vi "SRX_Config_Set Limit Travel Values.vi"(6 "Send Cmd Timout(ms)":u32, 8 "Error":errorcluster, 9 "Limits":T6 {"Soft"."REV"."Counts" format="%#.0f"; "Soft"."FWD"."Counts" format="%#.0f"}, 11 "PhoenixMotorControlDevRef":T1) -> (0 "Error Out":errorcluster, 3 "PhoenixMotorControlDevRef Out":T1)   [LabVIEW 2020]
uses:
  Shared Code/TypeDefs/Cluser_Limit Travel Config.ctl
  Shared Code/TypeDefs/Cluser_Hard Limits.ctl
  <vilib>/Rock Robotics/WPI/ThirdParty/Phoenix-LabVIEW/Motor Controller/Controls/CTRE_Phoenix_MotorControl_LimitSwitchNormal.ctl
  Shared Code/TypeDefs/Cluser_Config_Soft Limits.ctl
  Shared Code/TypeDefs/Cluser_Enable-Value I32.ctl
  <vilib>/Rock Robotics/WPI/MotorControl/WPI_MotorControlDeviceRef.ctl
  <vilib>/Rock Robotics/WPI/MotorControl/WPI_MotorControlType.ctl
  <vilib>/Rock Robotics/SystemInterfaces/DIO/FPGA_DIOPWMChannel.ctl
  <vilib>/Rock Robotics/WPI/PWM/WPI_PWMDeadband.ctl
  <vilib>/Rock Robotics/SystemInterfaces/DIO/FPGA_DIOChannel.ctl
  <vilib>/Rock Robotics/WPI/ThirdParty/Phoenix-LabVIEW/Motor Controller/Controls/CTRE_Phoenix_MotorControl_LimitSwitchSource_Local.ctl
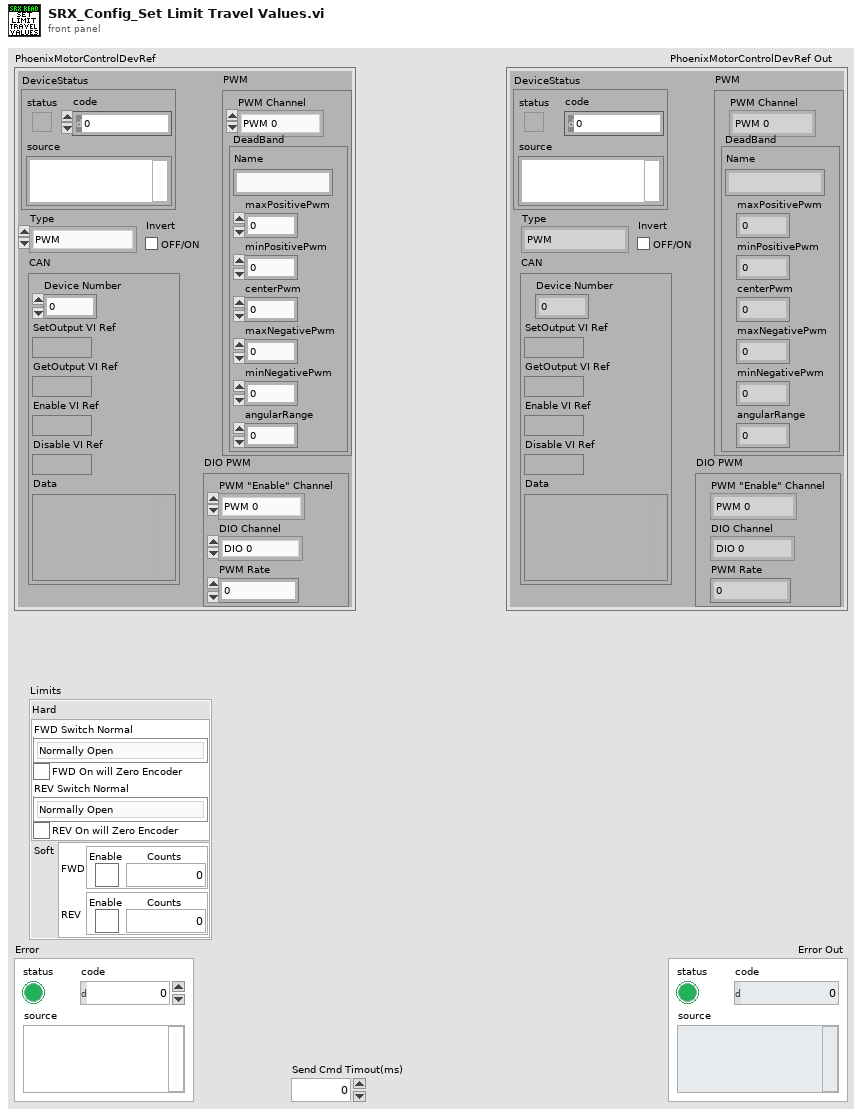
[diagram p1: front panel]
types:
  T1 = typedef "WPI_MotorControlDeviceRef.ctl" = cluster{"DeviceStatus":errorcluster, "Type":T2, "PWM":cluster{"PWM Channel":T3, "DeadBand":T4}, "CAN":cluster{"Device Number":u8, "SetOutput VI Ref":variant, "GetOutput VI Ref":variant, "Enable VI Ref":variant, "Disable VI Ref":variant, "Data":variant}, "Invert":bool, "DIO PWM":cluster{"PWM \"Enable\" Channel":T3, "DIOChannel":T5, "PWM Rate":dbl}}
  T2 = typedef "WPI_MotorControlType.ctl" = enum16{"PWM", "CAN", "DIO PWM"}
  T3 = typedef "FPGA_DIOPWMChannel.ctl" = enum8{"PWM 0", "PWM 1", "PWM 2", "PWM 3", "PWM 4", "PWM 5", "PWM 6", "PWM 7", "PWM 8", "PWM 9", "PWM MXP 0", "PWM MXP 1", "PWM MXP 2", "PWM MXP 3", "PWM MXP 4", "PWM MXP 5", "PWM MXP 6", "PWM MXP 7", "PWM MXP 8", "PWM MXP 9", "Invalid"}
  T4 = typedef "WPI_PWMDeadband.ctl" = cluster{"Name":string, "maxPositivePwm":i32, "minPositivePwm":i32, "centerPwm":i32, "maxNegativePwm":i32, "minNegativePwm":i32, "angularRange":u16}
  T5 = typedef "FPGA_DIOChannel.ctl" = enum8{"DIO 0", "DIO 1", "DIO 2", "DIO 3", "DIO 4", "DIO 5", "DIO 6", "DIO 7", "DIO 8", "DIO 9", "DIO MXP 0", "DIO MXP 1", "DIO MXP 2", "DIO MXP 3", "DIO MXP 4", "DIO MXP 5", "DIO MXP 6", "DIO MXP 7", "DIO MXP 8", "DIO MXP 9", "DIO MXP 10", "DIO MXP 11", "DIO MXP 12", "DIO MXP 13", "DIO MXP 14", "DIO MXP 15", "SPI Port CS1", "SPI Port CS2", "SPI Port CS3", "SPI Port MISO", "SPI Port MOSI", "Invalid"}
  T6 = typedef "Cluser_Limit Travel Config.ctl" = cluster{"Hard":T7, "Soft":T9}
  T7 = typedef "Cluser_Hard Limits.ctl" = cluster{"FWD Switch Normal":T8, "FWD On will Zero Encoder ":bool, "REV Switch Normal":T8, "REV On will Zero Encoder ":bool}
  T8 = typedef "CTRE_Phoenix_MotorControl_LimitSwitchNormal.ctl" = enum16{"Normally Open", "Normally Closed", "Disabled"}
  T9 = typedef "Cluser_Config_Soft Limits.ctl" = cluster{"FWD":T10, "REV":T10}
  T10 = typedef "Cluser_Enable-Value I32.ctl" = cluster{"Enable":bool, "Counts":i32}
  T11 = typedef "CTRE_Phoenix_MotorControl_LimitSwitchSource_Local.ctl" = enum16{"Feedback Connector", "Remote Talon SRX", "Remote CANifier", "Deactivated"}
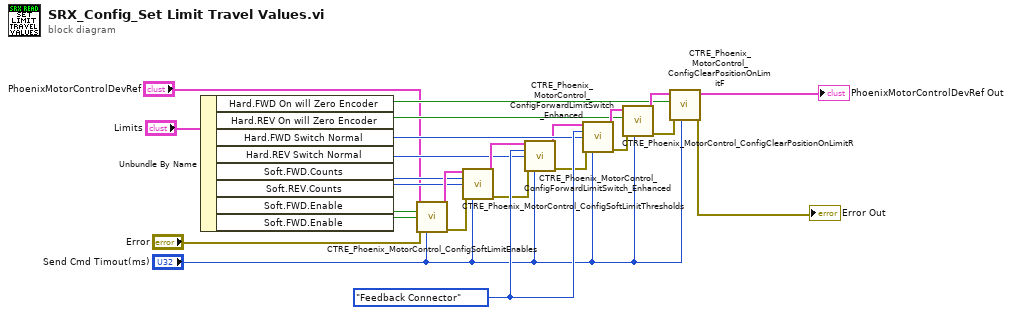
[diagram p0: block diagram]
diagram:
  w16 = CTRE_Phoenix_MotorControl_LimitSwitchSource_Local."Feedback Connector" ("Limit Switch Source")
  n1 = Unbundle By Name("Limits") -> ("Hard.FWD On will Zero Encoder"=w5:bool, "Hard.REV On will Zero Encoder"=w8:bool, "Hard.FWD Switch Normal"=w14:T8, "Hard.REV Switch Normal"=w15:T8, "Soft.FWD.Counts"=w19:i32, "Soft.REV.Counts"=w18:i32, "Soft.FWD.Enable"=w24:bool, "Soft.FWD.Enable"=w23:bool)
  n2 = call <vilib>:"CTRE_Phoenix_MotorControl_ConfigSoftLimitEnables.vi"("PhoenixMotorControlDevRef"="PhoenixMotorControlDevRef", "Forward Soft Limit Enable"=w24, "Reverse Soft Limit Enable"=w23, "error in (no error)"="Error", "timeoutMs"="Send Cmd Timout(ms)") -> ("PhoenixMotorControlDevRef"=w20:T1, "error out"=w21:errorcluster)  [unwired: 9 in]
  n3 = call <vilib>:"CTRE_Phoenix_MotorControl_ConfigSoftLimitThresholds.vi"("PhoenixMotorControlDevRef"=w20, "Forward Soft Limit"=w19, "Reverse Soft Limit"=w18, "error in (no error)"=w21, "timeoutMs"="Send Cmd Timout(ms)") -> ("PhoenixMotorControlDevRef"=w17:T1, "error out"=w12:errorcluster)  [unwired: 9 in]
  n4 = call <vilib>:"CTRE_Phoenix_MotorControl_ConfigForwardLimitSwitch_Enhanced.vi"("PhoenixMotorControlDevRef"=w17, "Limit Switch Source"=w16, "NormallyOpenOrClosed"=w15, "error in (no error)"=w12, "timeoutMs"="Send Cmd Timout(ms)") -> ("PhoenixMotorControlDevRef"=w11:T1, "error out"=w13:errorcluster)  [unwired: 9 in]
  n5 = call <vilib>:"CTRE_Phoenix_MotorControl_ConfigForwardLimitSwitch_Enhanced.vi"("PhoenixMotorControlDevRef"=w11, "Limit Switch Source"=w16, "NormallyOpenOrClosed"=w14, "error in (no error)"=w13, "timeoutMs"="Send Cmd Timout(ms)") -> ("PhoenixMotorControlDevRef"=w9:T1, "error out"=w10:errorcluster)  [unwired: 9 in]
  n6 = call <vilib>:"CTRE_Phoenix_MotorControl_ConfigClearPositionOnLimitR.vi"("timeoutMs"="Send Cmd Timout(ms)", "error in (no error)"=w10, "Clear Position On Limit R"=w8, "PhoenixMotorControlDevRef"=w9) -> ("error out"=w7:errorcluster, "PhoenixMotorControlDevRef"=w6:T1)  [unwired: 6 in]
  n7 = call <vilib>:"CTRE_Phoenix_MotorControl_ConfigClearPositionOnLimitF.vi"("timeoutMs"="Send Cmd Timout(ms)", "error in (no error)"=w7, "Clear Position On Limit F"=w5, "PhoenixMotorControlDevRef"=w6) -> ("error out"=→"Error Out":errorcluster, "PhoenixMotorControlDevRef"=→"PhoenixMotorControlDevRef Out":T1)  [unwired: 6 in]
